vi "Count.vi"(1 "TestSuite In":refnum<class "TestSuite.lvclass">) -> (0 "Count":i32)   [LabVIEW 2019, in "TestSuite.lvclass"]
doc: "Counts the number of test cases that will be run by this test."
uses:
  TestSuite.lvclass
  TestSuite.lvclass/TestSuite.ctl
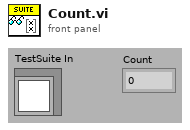
[diagram p1: front panel]
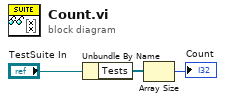
[diagram p0: block diagram]
diagram:
  n1 = Unbundle By Name("TestSuite In") -> ("Tests"=w2:refnum<class "TestCase.lvclass">[])
  n2 = Array Size(array=w2) -> (size(s)=→"Count":i32)
